vi "Set_Reset.vi"(11 "board PF":bool[](array[boolean])) -> (1 "数值":i16, 2 "数组":string[](array[string]), 3 "字符串":string)   [LabVIEW 2018]
uses:
  Global.vi
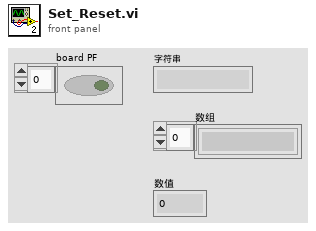
[diagram p1: front panel]
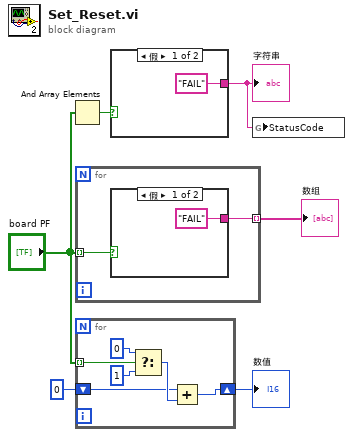
[diagram p0: block diagram]
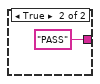
[diagram p2: hidden frame]
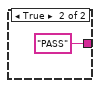
[diagram p3: hidden frame]
diagram:
  n1 = And Array Elements(Boolean array="board PF") -> (logical AND=w1:bool)
  n2 = for {
    tunnel: "board PF" -> [w8] mode=indexing
    tunnel: [w7] -> w2 mode=indexing
    n3 = case shown="假" w8 {
      tunnel: ["FAIL" "PASS" ("字符串")] -> w7
      frame False {
      }
      frame True {
      }
    }
  }
  "数组" <- w2
  n4 = for {
    shift-right: [w11] -> w3
    shift-left: i16 0 -> [w12]
    tunnel: "board PF" -> [w13] mode=indexing
    n5 = Select(t=i16 0 ("精度(6)"), s=w13, f=i16 1 ("精度(6)")) -> (s? t:f=w14:i16)
    n6 = Add(x=w12, y=w14) -> (x+y=w11:i16)
  }
  "数值" <- w3
  n7 = case shown="假" w1 {
    tunnel: ["FAIL" "PASS" ("字符串")] -> w5
    frame False {
    }
    frame True {
    }
  }
  "字符串" <- w5
  n8 = global write "Global.vi" "StatusCode"(w5) -> ()
